vi "cbm.vi"() -> ()   [LabVIEW 2017]
uses:
  typedefs/stagestates.ctl
  typedefs/stagequeue.ctl
  typedefs/Camqueue.ctl
  typedefs/Camstates.ctl
  <vilib>/Analysis/NI_AALBase.lvlib
  <vilib>/Utility/miscctls.llb/LVMinMaxIncTypeDef.ctl
panel:
  out "white level":u16
  out "black level":u16
  out "Ranges":T2
  out "total time":u32
  out "average time per step":dbl
  out "start time":u32
  out "Stack Folder":path
  in  "Image path used":path
  in  "Save next image":bool
  out "Image":u16[][](graph)
  in  "Live Update":bool
  out "Cam ready":bool
  out "Scan points":dbl[](array[numeric])
  in  "Get mean image button":bool
  in  "Get random stack":bool
  in  "abort button":bool
  in  "Get Speckle Stack button":bool
  in  "stop button":bool
  in  "Stage position":dbl(slide) scale=-3000.0..3000.0
  in  "Tab Control":enum32{"Stage", "Camera"}(tab)
  in  "Folder Name":string
  in  "Base path":path=path "D:/Jean-Claude/180614 clem uzh"
  in  "Speckle Stack Settings":T3={"Start Position[µm]"=-150.0, "Final Position[µm]"=150.0, "Number of frames"=100} {"Number of frames" min=2; "Final Position[µm]" min=-6000.0 max=6000.0; "Start Position[µm]" min=-6000.0 max=6000.0}
  in  "Zero Ch2":bool
  out "Stage State":T4=enum."Init"
  out "Stage initialized":bool
  out "stack folder":path
  in  "settling time":u32=20
  out "size stage queue":i32
  in  "ChangeCamSettings":bool
  out "Current Settings":T5
  out "Camera Details":T6
  out "Cam state":T7
  in  "Camera index":u32
  out "Initialized":bool
  in  "use cam":bool=TRUE
  in  "input cluster":T8={"binning"=0.0, "exp. time[ms]"=100.0, "v. offset"=0, "h. offset"=0, "width"=3000, "height"=1024} {"binning" min=0.0 max=2.0 step=1.0; "v. offset" max=2048 step=4; "h. offset" max=2048 step=4; "width" max=2048 step=4; "height" max=2048 step=4}
  out "size cam queue":i32
  out "Histogram":T9(graph)
  in  "Black and White levels":cluster{u16, u16}(slide)={0, 255} scale=0.0..65535.0
  in  "scale exp":bool
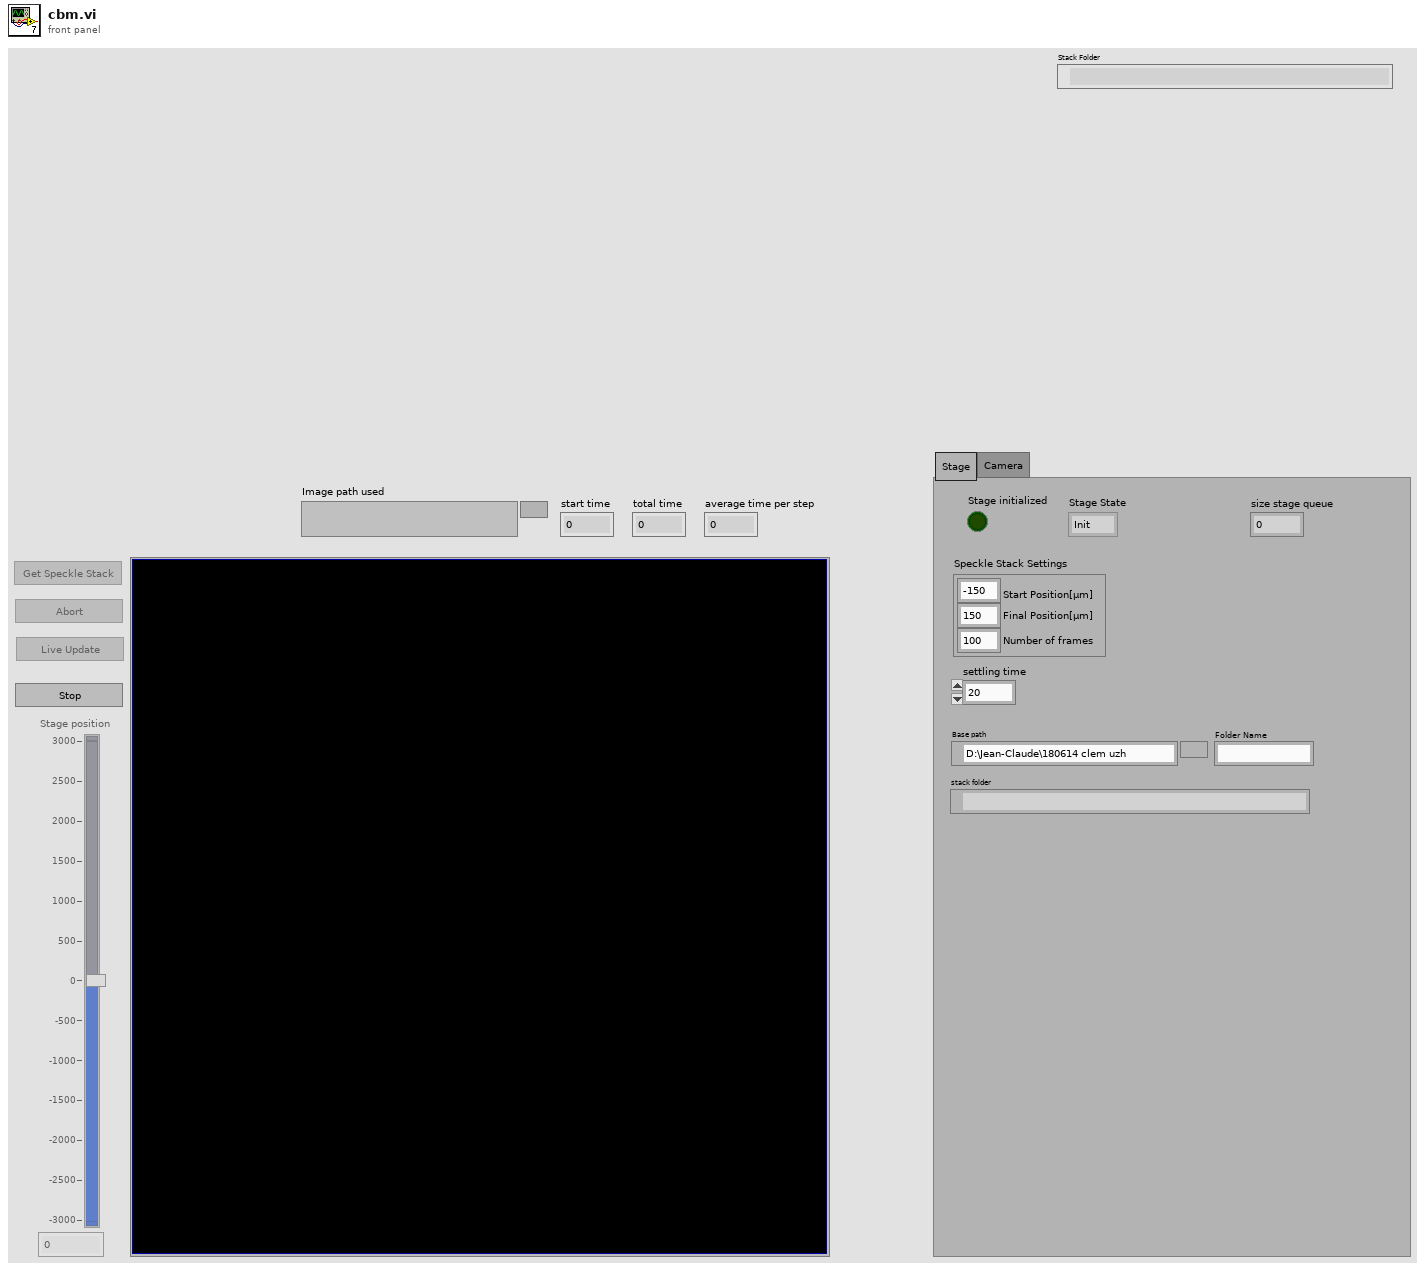
[diagram p1: front panel]
types:
  T1 = typedef "LVMinMaxIncTypeDef.ctl" = cluster{"Minimum":dbl, "Maximum":dbl, "Increment":dbl}
  T2 = cluster{"HorPosRange":T1, "VertPosRange":T1, "WidthRange":T1, "HeightRange":T1}
  T3 = cluster{"Start Position[µm]":dbl, "Final Position[µm]":dbl, "Number of frames":u32}
  T4 = typedef "stagestates.ctl" = enum16{"zero", "move", "Init", "idle", "init scan", "scan", "finish scan", "error", "stop"}
  T5 = cluster{"binning":dbl, "exposure time[s]":dbl, "v. offset":dbl, "h. offset":dbl, "width":dbl, "height":dbl}
  T6 = cluster{"Model":string, "Camera ID":string, "Firmware":string}
  T7 = typedef "Camstates.ctl" = enum16{"Intitializing", "idling", "change settings", "take snapshot", "error", "stop"}
  T8 = cluster{"binning":dbl, "exp. time[ms]":dbl, "v. offset":u32, "h. offset":u32, "width":u32, "height":u32}
  T9 = cluster{"X Values":dbl[], "Histogram: h(x)":i32[]}
  T10 = typedef "Camqueue.ctl" = enum16{"initialize camera", "Take snapshot", "Change settings", "Stop", "Scan"}
  T11 = typedef "stagequeue.ctl" = enum16{"idle", "initialize stage", "move ch2", "zero ch2", "Scan", "Stop"}
  T12 = cluster{"posX":i32, "posY":i32, "Width":i32, "height":i32}
  T13 = typedef "imagedata.ctl" = cluster{"image type":i32, "image depth":i32, "image":u8[], "mask":u8[], "colors":u32[], "Rectangle":cluster{"left":i16, "top":i16, "right":i16, "bottom":i16}}
  T14 = enum8{"Enabled", "Disabled", "Disabled and Grayed Out"}
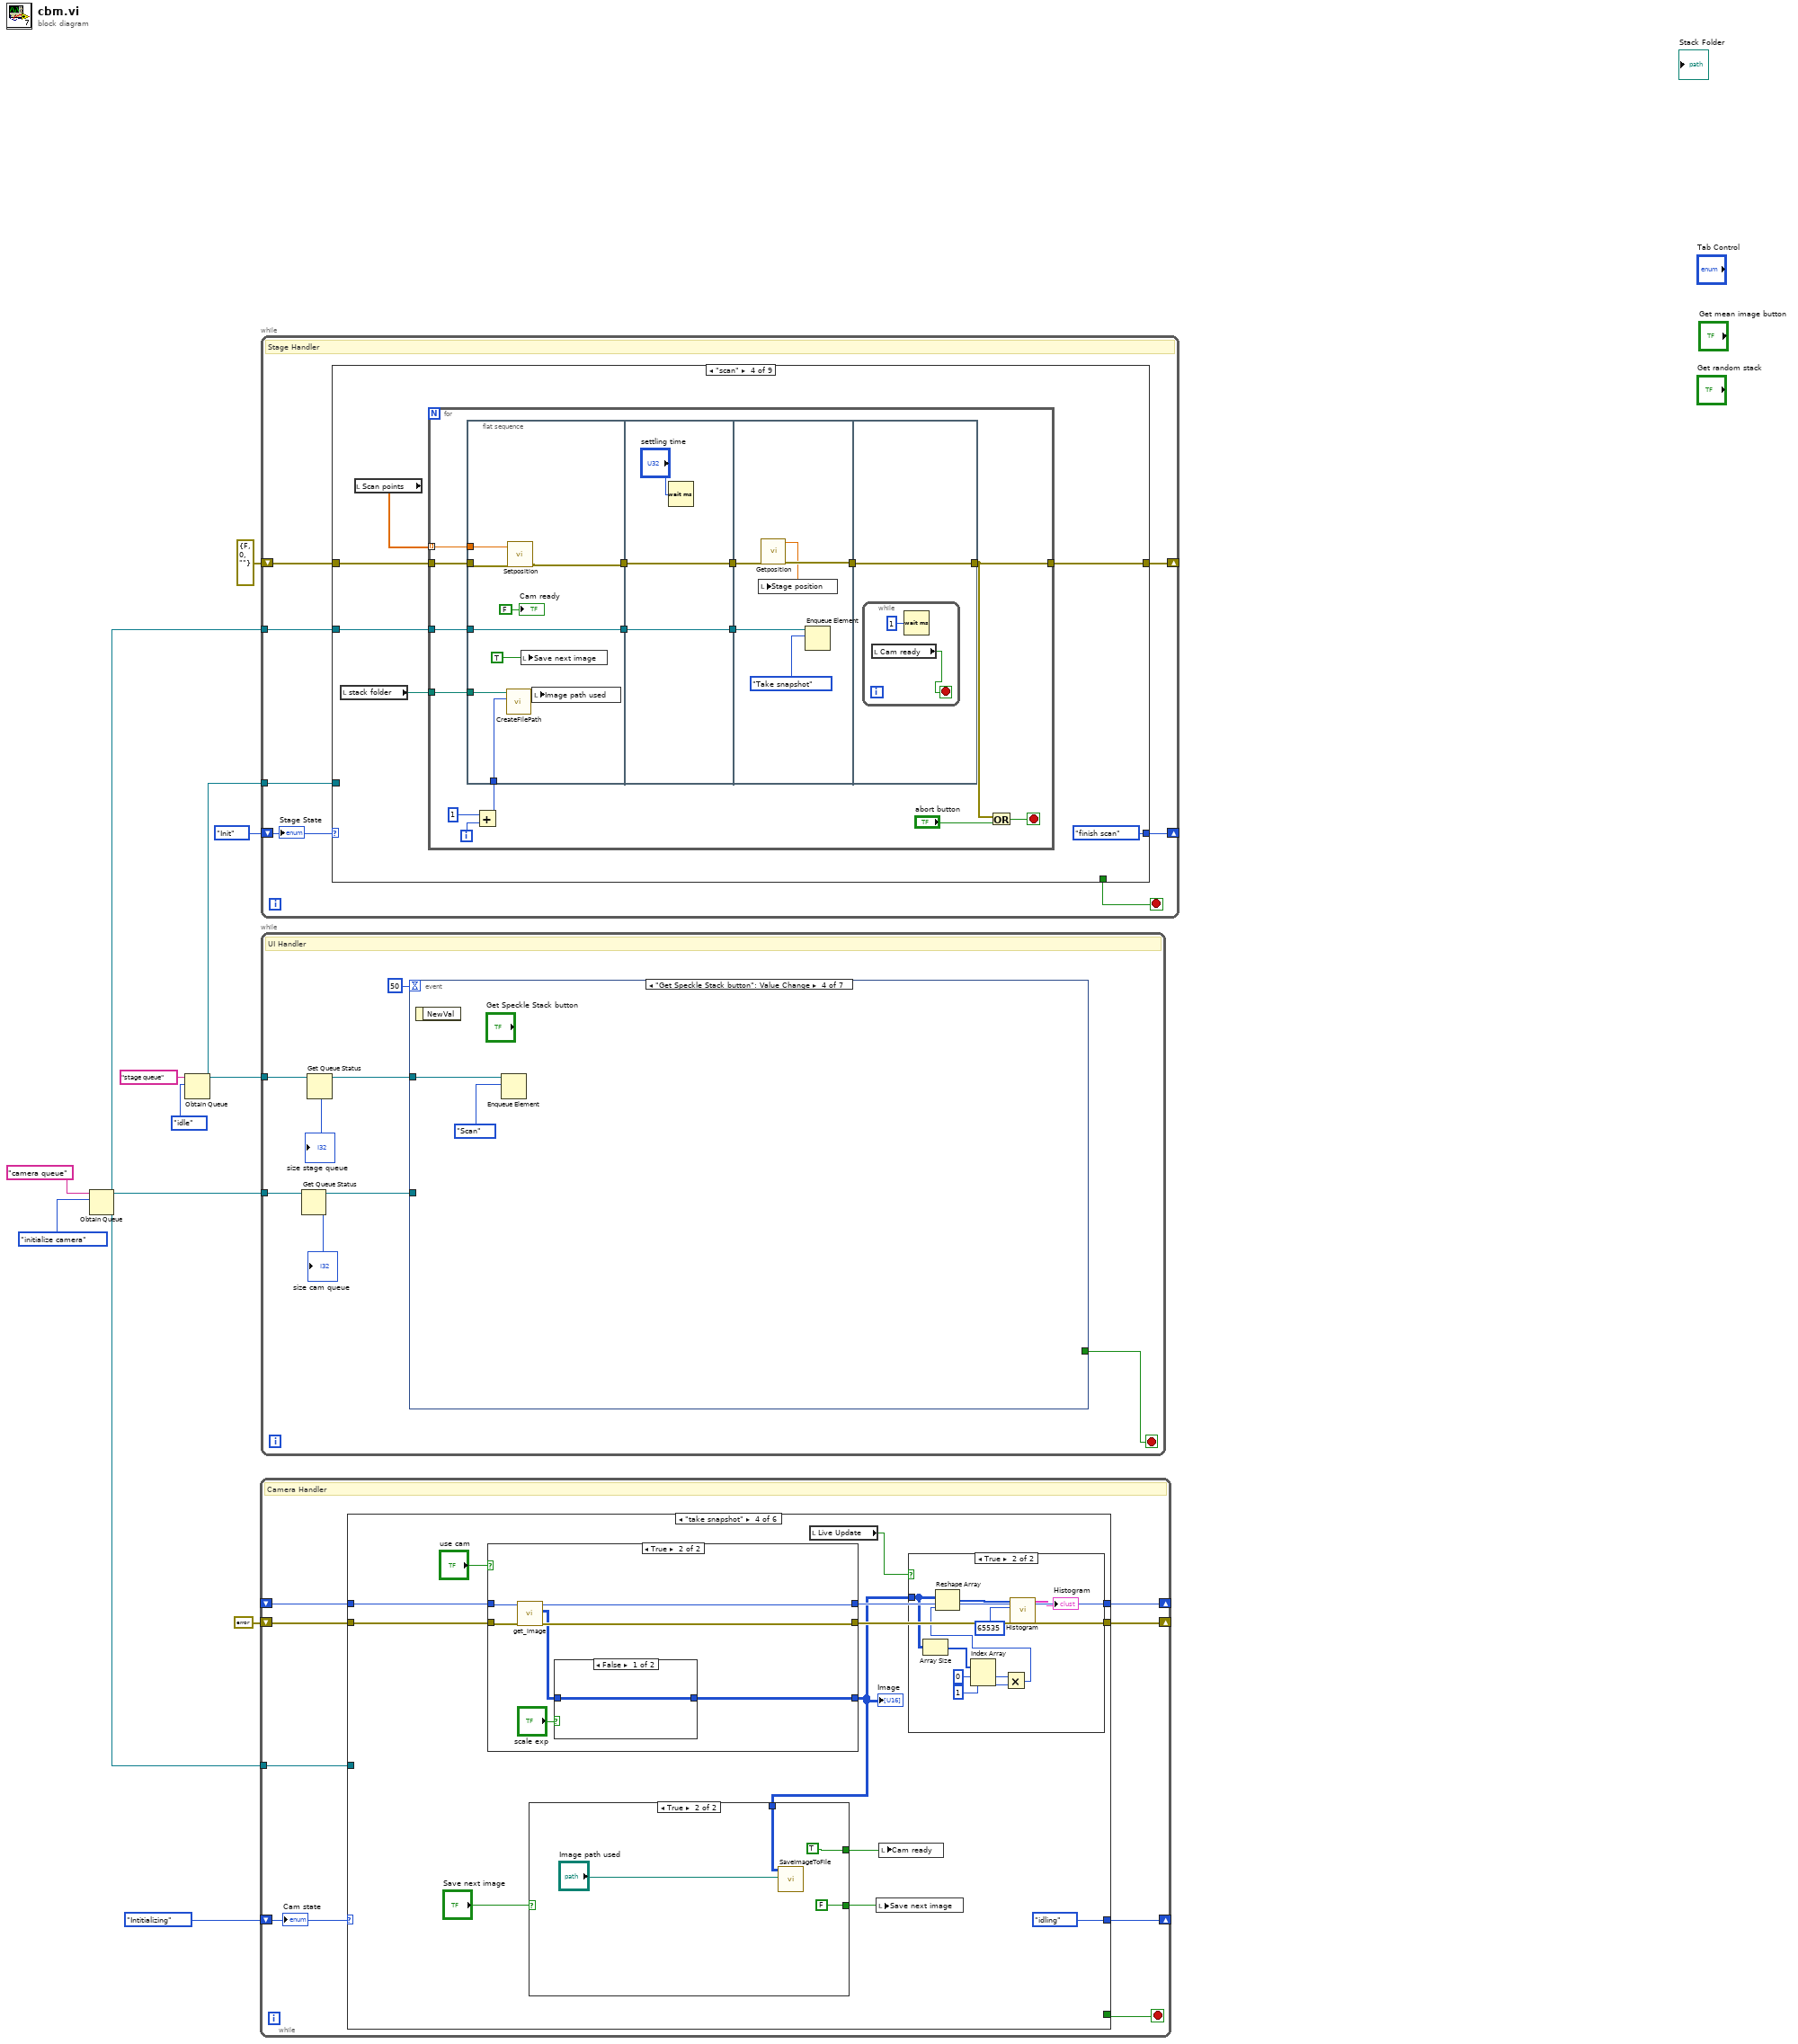
[diagram p0: block diagram]
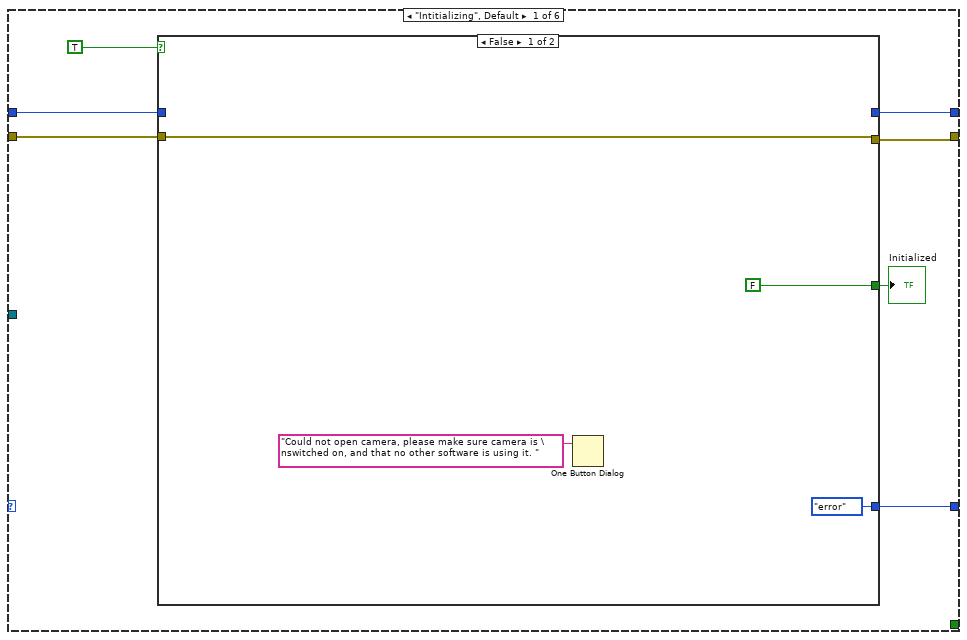
[diagram p2: hidden frame]
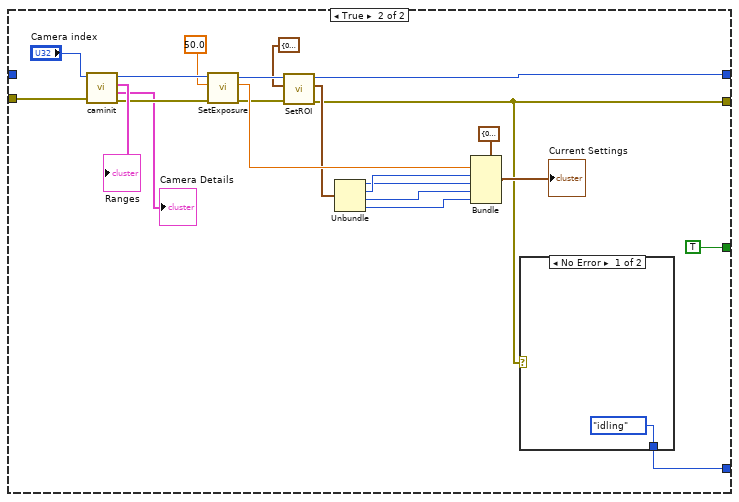
[diagram p3: hidden frame]
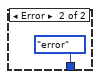
[diagram p4: hidden frame]
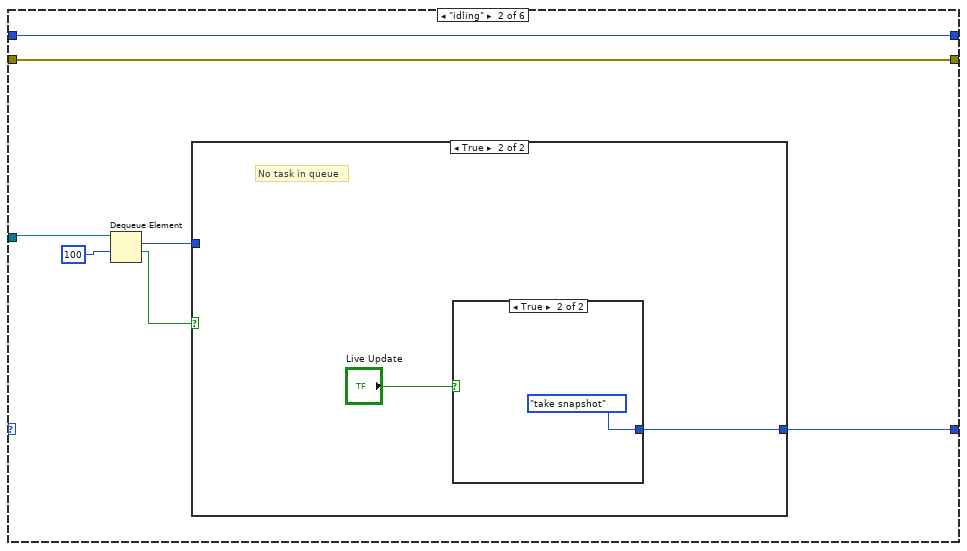
[diagram p5: hidden frame]
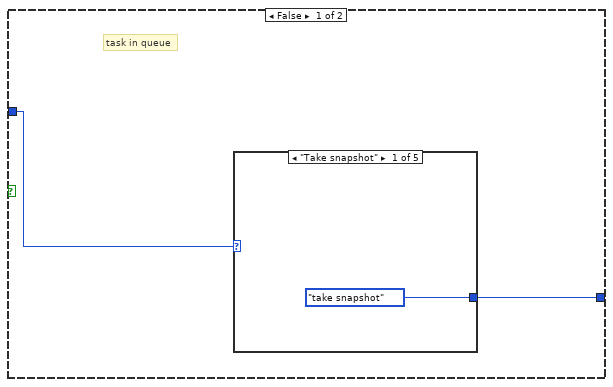
[diagram p6: hidden frame]
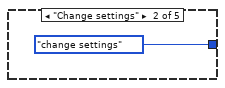
[diagram p7: hidden frame]
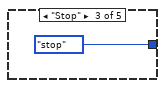
[diagram p8: hidden frame]
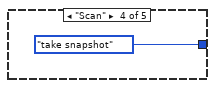
[diagram p9: hidden frame]
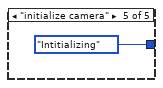
[diagram p10: hidden frame]
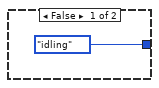
[diagram p11: hidden frame]
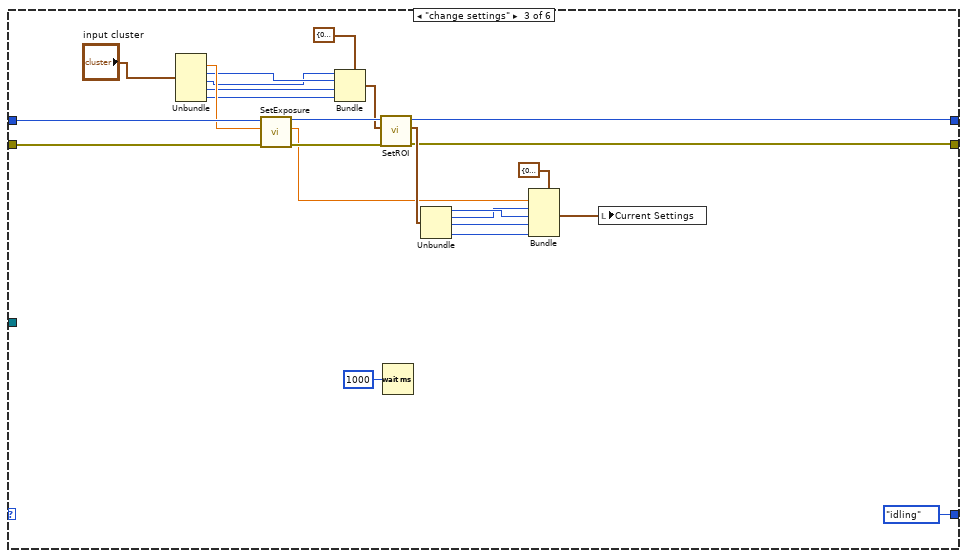
[diagram p12: hidden frame]
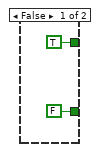
[diagram p14: hidden frame]
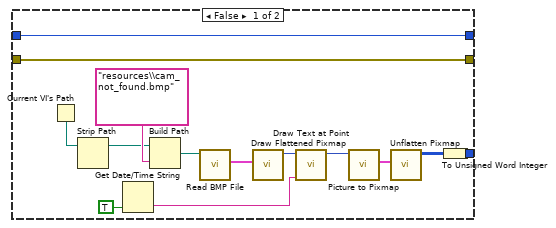
[diagram p15: hidden frame]
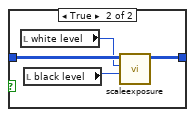
[diagram p16: hidden frame]
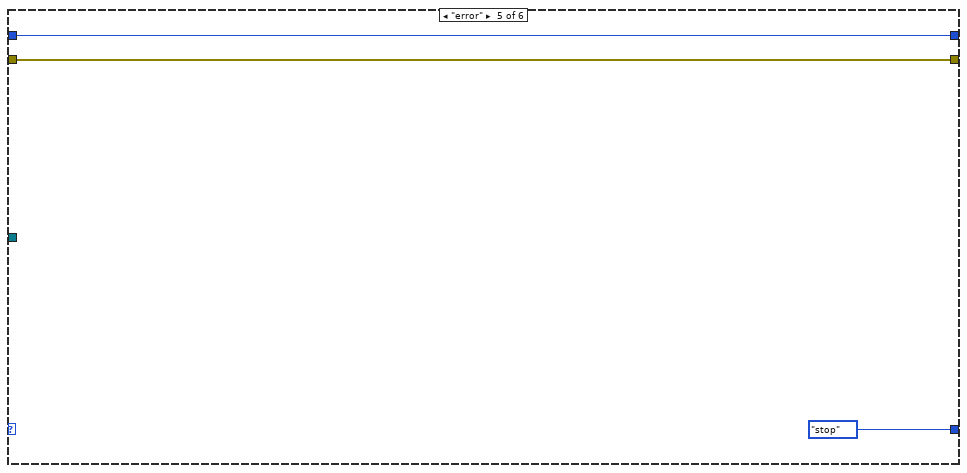
[diagram p17: hidden frame]
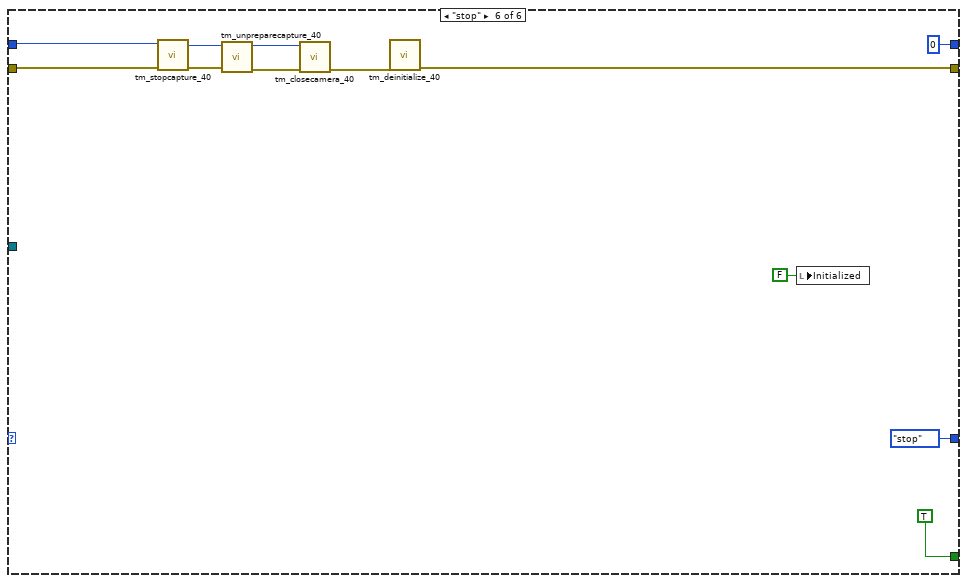
[diagram p18: hidden frame]
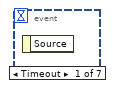
[diagram p19: hidden frame]
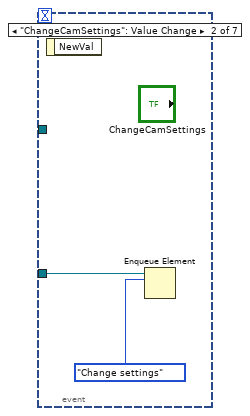
[diagram p20: hidden frame]
diagram:
  n1 = Obtain Queue(name (unnamed)="camera queue", element data type=Camqueue."initialize camera") -> (queue out=w1:refnum<queue>)  [unwired: 3 in, 2 out]
  n2 = Obtain Queue(name (unnamed)="stage queue", element data type=stagequeue."idle") -> (queue out=w5:refnum<queue>)  [unwired: 3 in, 2 out]
  n3 = while {
    tunnel: w1 -> [w11]
    shift-right: [w14] -> _
    shift-left: errorcluster {"status"=FALSE, "code"=0, "source"=""} ("error in (no error)") -> [w16]
    shift-right: [w15] -> _
    shift-left: _ -> [w12]
    shift-right: [w13] -> _
    shift-left: Camstates."Intitializing" -> [w18]
    stop <- w17 stop-if-true
    # "Camera Handler"
    n4 = case shown="\"take snapshot\"" w18 {
      tunnel: [_ _ _ _ _ TRUE] -> w17
      tunnel: w16 -> [w20 w59 w90 w104 w150 w160]
      tunnel: [w25 w60 w72 w103 w149 u32 0 ("Handle out")] -> w15
      tunnel: [w19 w59 w73 w102 w150 w156] -> w14
      tunnel: [w23 w54 Camstates."idling" Camstates."idling" Camstates."stop" Camstates."stop"] -> w13
      tunnel: w12 -> [w21 w60 w92 w105 w149 w152]
      tunnel: w11 -> [_ w58 _ _ _ _]
      frame "Intitializing", Default {
        n5 = case shown="False" TRUE {
          tunnel: [_ w40] -> w25
          tunnel: [FALSE ("Initialized") TRUE ("Initialized")] -> w24
          tunnel: [Camstates."error" w50] -> w23
          tunnel: w21 -> [_ _]
          tunnel: w20 -> [w26 w43]
          tunnel: [w26 w32] -> w19
          frame False {
            n6 = One Button Dialog(message="Could not open camera, please make sure camera is \nswitched on, and that no other software is using it. ") -> ()  [unwired: 1 in, 1 out]
          }
          frame True {
            n7 = call "caminit.vi"("error in (no error)"=w43, "Camera Index"="Camera index") -> ("error out"=w44:errorcluster, "Cam Info"=→"Camera Details":T6, "Ranges"=→"Ranges":T2, "Handle out"=w47:u32)  [unwired: 5 in]
            n8 = call "SetExposure.vi"("error in (no error)"=w44, "Exposure[ms]"=50.0, "Handle in"=w47) -> ("error out"=w33:errorcluster, "exposure"=w45:dbl, "Handle out"=w42:u32)  [unwired: 4 in, 1 out]
            n9 = call "SetROI.vi"("error in (no error)"=w33, "SizeIn"=T12 {"posX"=0, "posY"=0, "Width"=2048, "height"=2048}, "Handle in"=w42) -> ("error out"=w32:errorcluster, "sizeout"=w38:T12, "Handle out"=w40:u32)  [unwired: 5 in]
            n10 = Unbundle(w38) -> ("posX"=w36:i32, "posY"=w37:i32, "Width"=w35:i32, "height"=w34:i32)
            n11 = Bundle(cluster=T5 {"binning"=0.0, "exposure time[s]"=0.0, "v. offset"=0.0, "h. offset"=0.0, "width"=0.0, "height"=0.0} ("Current Settings"), "exposure time[s]"=w45, "v. offset"=w37, "h. offset"=w36, "width"=w35, "height"=w34) -> (→"Current Settings":T5)  [unwired: 1 in]
            n12 = case shown="No Error" w32 {
              tunnel: [Camstates."idling" Camstates."error"] -> w50
              frame No Error {
              }
              frame Error {
              }
            }
          }
        }
        "Initialized" <- w24
      }
      frame "idling" {
        n13 = Dequeue Element(queue=w58, timeout in ms (-1)=100) -> (element=w55:T10, timed out?=w56:bool)  [unwired: 1 in, 2 out]
        n14 = case shown="True" w56 {
          tunnel: w55 -> [w62 _]
          tunnel: [w61 w68] -> w54
          frame False {
            # "task in queue"
            n15 = case shown="\"Take snapshot\"" w62 {
              tunnel: [Camstates."take snapshot" Camstates."change settings" Camstates."stop" Camstates."take snapshot" Camstates."Intitializing"] -> w61
              frame "Take snapshot" {
              }
              frame "Change settings" {
              }
              frame "Stop" {
              }
              frame "Scan" {
              }
              frame "initialize camera" {
              }
            }
          }
          frame True {
            # "No task in queue"
            n16 = case shown="True" "Live Update" {
              tunnel: [Camstates."idling" Camstates."take snapshot"] -> w68
              frame False {
              }
              frame True {
              }
            }
          }
        }
      }
      frame "change settings" {
        n17 = Unbundle("input cluster") -> ("exp. time[ms]"=w91:dbl, "v. offset"=w85:u32, "h. offset"=w84:u32, "width"=w83:u32, "height"=w82:u32)  [unwired: 1 out]
        n18 = call "SetExposure.vi"("error in (no error)"=w90, "Exposure[ms]"=w91, "Handle in"=w92) -> ("error out"=w88:errorcluster, "exposure"=w78:dbl, "Handle out"=w89:u32)  [unwired: 4 in, 1 out]
        n19 = Bundle(cluster=T12 {"posX"=0, "posY"=0, "Width"=0, "height"=0} ("SizeIn"), "posX"=w84, "posY"=w85, "Width"=w83, "height"=w82) -> (w86:T12)
        n20 = call "SetROI.vi"("error in (no error)"=w88, "SizeIn"=w86, "Handle in"=w89) -> ("error out"=w73:errorcluster, "sizeout"=w79:T12, "Handle out"=w72:u32)  [unwired: 5 in]
        n21 = Wait (ms)(milliseconds to wait=u32 1000) -> ()  [unwired: 1 out]
        n22 = Unbundle(w79) -> ("posX"=w77:i32, "posY"=w76:i32, "Width"=w75:i32, "height"=w74:i32)
        n23 = Bundle(cluster=T5 {"binning"=0.0, "exposure time[s]"=0.0, "v. offset"=0.0, "h. offset"=0.0, "width"=0.0, "height"=0.0} ("Current Settings"), "exposure time[s]"=w78, "v. offset"=w76, "h. offset"=w77, "width"=w75, "height"=w74) -> (w80:T5)  [unwired: 1 in]
        n24 = local write "Current Settings"(w80) -> ()
      }
      frame "take snapshot" {
        n25 = case shown="True" "use cam" {
          tunnel: w104 -> [w132 w143]
          tunnel: [w132 w142] -> w102
          tunnel: [w131 w140] -> w103
          tunnel: w105 -> [w131 w141]
          tunnel: [w123 w138] -> w96
          frame False {
            n26 = Current VI's Path() -> (path=w136:path)
            n27 = Strip Path(path=w136) -> (stripped path=w134:path)  [unwired: 1 out]
            n28 = Get Date/Time String(want seconds? (F)=TRUE) -> (time string=w128:string)  [unwired: 2 in, 1 out]
            n29 = Build Path(base path=w134, name or relative path="resources\\cam_not_found.bmp") -> (appended path=w133:path)
            n30 = call <vilib>:"Read BMP File.vi"("path to BMP file"=w133) -> ("image data"=w130:T13)  [unwired: 8 in, 2 out]
            n31 = call <vilib>:"Draw Flattened Pixmap.vi"("image data"=w130) -> ("new picture"=w129:picture)  [unwired: 8 in]
            n32 = call <vilib>:"Draw Text at Point.vi"("text"=w128, "picture"=w129) -> ("new picture"=w127:picture)  [unwired: 8 in, 1 out]
            n33 = call <vilib>:"Picture to Pixmap.vi"("picture"=w127) -> ("image data"=w126:T13)  [unwired: 9 in, 1 out]
            n34 = call <vilib>:"Unflatten Pixmap.vi"("image data"=w126) -> ("24-bit pixmap"=w124:u32[][])  [unwired: 4 in, 6 out]
            n35 = To Unsigned Word Integer(number=w124) -> (unsigned 16bit integer=w123:u16[][])
          }
          frame True {
            n36 = call "get_image.vi"("error in (no error)"=w143, "Handle in"=w141) -> ("error out"=w142:errorcluster, "Data"=w139:u16[][], "Handle out"=w140:u32)  [unwired: 7 in]
            n37 = case shown="False" "scale exp" {
              tunnel: w139 -> [w144 w148]
              tunnel: [w144 w147] -> w138
              frame False {
              }
              frame True {
                n38 = local read "white level"() -> (w146:u16)
                n39 = local read "black level"() -> (w145:u16)
                n40 = call "scaleexposure.vi"("black"=w145, "white"=w146, "image in"=w148) -> ("image out"=w147:u16[][])  [unwired: 8 in]
              }
            }
          }
        }
        "Image" <- w96
        n41 = case shown="True" "Save next image" {
          tunnel: [FALSE ("Save next image") FALSE ("Save next image")] -> w100
          tunnel: [TRUE TRUE] -> w99
          tunnel: w96 -> [_ w119]
          frame False {
          }
          frame True {
            n42 = call "SaveImageToFile.vi"("File Path"="Image path used", "Image Pixels (U16)"=w119) -> ()  [unwired: 9 in, 1 out]
          }
        }
        n43 = local read "Live Update"() -> (w97:bool)
        n44 = local write "Save next image"(w100) -> ()
        n45 = local write "Cam ready"(w99) -> ()
        n46 = case shown="True" w97 {
          tunnel: w96 -> [_ w115]
          frame False {
          }
          frame True {
            n47 = Array Size(array=w115) -> (size(s)=w112:i32[])
            n48 = Index Array(array=w112, index #1=0 ("index"), index #2=1 ("index")) -> (element #1=w111:i32, element #2=w110:i32)
            n49 = Multiply(x=w111, y=w110) -> (x*y=w109:i32)
            n50 = Reshape Array(w115, w109) -> (w116:u16[])
            n51 = call <vilib>:"Histogram.vi"("intervals"=65535, "X"=w116) -> ("Histogram Graph"=→"Histogram":T9)  [unwired: 6 in, 3 out]
          }
        }
      }
      frame "error" {
      }
      frame "stop" {
        n52 = call <userlib>:"tm_stopcapture_40.vi"("error in (no error)"=w160, "Handle in"=w152) -> ("error out"=w159:errorcluster, "Handle out"=w153:u32)  [unwired: 8 in]
        n53 = call <userlib>:"tm_unpreparecapture_40.vi"("error in (no error)"=w159, "Handle in"=w153) -> ("error out"=w158:errorcluster, "Handle out"=w154:u32)  [unwired: 8 in]
        n54 = call <userlib>:"tm_closecamera_40.vi"("error in (no error)"=w158, "Handle in"=w154) -> ("error out"=w157:errorcluster)  [unwired: 9 in]
        n55 = call <userlib>:"tm_deinitialize_40.vi"("error in (no error)"=w157) -> ("error out"=w156:errorcluster)  [unwired: 10 in]
        n56 = local write "Initialized"(FALSE ("Initialized")) -> ()
      }
    }
    "Cam state" <- w18
  }
  n57 = while {
    shift-right: [w169] -> _
    shift-left: stagestates."Init" -> [w170]
    shift-right: [w168] -> _
    shift-left: errorcluster {"status"=FALSE, "code"=0, "source"=""} ("error out") -> [w167]
    tunnel: w5 -> [w165]
    tunnel: w1 -> [w164]
    stop <- w166 stop-if-true
    # "Stage Handler"
    n58 = case shown="\"scan\"" w170 {
      tunnel: [w174 w187 stagestates."scan" stagestates."finish scan" stagestates."idle" stagestates."Init" stagestates."stop" stagestates."idle" stagestates."idle"] -> w169
      tunnel: [w171 w184 w221 w235 w281 w286 w297 w302 w306] -> w168
      tunnel: w167 -> [w172 w185 w221 w236 w281 w289 w298 w303 w306]
      tunnel: [FALSE FALSE FALSE _ _ _ TRUE _ _] -> w166
      tunnel: w165 -> [_ w191 _ _ _ _ _ _ _]
      tunnel: w164 -> [_ _ _ w234 _ _ _ _ _]
      frame "Init", Default {
        n59 = call "init.vi"("error in"=w172, "Controller S/N"="118032250") -> ("error out"=w171:errorcluster)  [unwired: 9 in]
        n60 = case shown="No Error" w171 {
          tunnel: [stagestates."error" stagestates."idle"] -> w174
          tunnel: [FALSE ("Stage initialized") TRUE ("Stage initialized")] -> w176
          frame Error {
            n61 = Wait (ms)(milliseconds to wait=u32 10000) -> ()  [unwired: 1 out]
          }
          frame No Error {
            w180 = T14."Enabled" ("Disabled")
            n62 = property on="Stage position" class="Slide (strict)"("DisabledEnum"=w180) -> ()  [unwired: 2 in, 2 out]
            n63 = property on="Get Speckle Stack button" class="Bool"("DisabledEnum"=w180) -> ()  [unwired: 2 in, 2 out]
            n64 = property on="Get mean image button" class="Bool"("DisabledEnum"=w180) -> ()  [unwired: 2 in, 2 out]
            n65 = property on="Get random stack" class="Bool"("DisabledEnum"=w180) -> ()  [unwired: 2 in, 2 out]
            n66 = property on="abort button" class="Bool"("DisabledEnum"=w180) -> ()  [unwired: 2 in, 2 out]
            n67 = property on="Live Update" class="Bool (strict)"("DisabledEnum"=w180) -> ()  [unwired: 2 in, 2 out]
          }
        }
        "Stage initialized" <- w176
      }
      frame "idle" {
        n68 = Dequeue Element(queue=w191, timeout in ms (-1)=20) -> (element=w189:T11, timed out?=w188:bool)  [unwired: 1 in, 2 out]
        n69 = case shown="True" w188 {
          tunnel: w189 -> [w194 _]
          tunnel: [w193 stagestates."idle"] -> w186
          frame False {
            # "Queue not empty"
            n70 = case shown="\"zero ch2\"" w194 {
              tunnel: [stagestates."idle" stagestates."Init" stagestates."move" stagestates."zero" stagestates."init scan" stagestates."stop"] -> w193
              frame "idle", Default {
              }
              frame "initialize stage" {
              }
              frame "move ch2" {
              }
              frame "zero ch2" {
              }
              frame "Scan" {
              }
              frame "Stop" {
              }
            }
          }
          frame True {
            # "Queue empty"
          }
        }
        n71 = call "Getposition.vi"("error in"=w185) -> ("error out"=w184:errorcluster, "Position[µm]"=w183:dbl)  [unwired: 9 in]
        n72 = case shown="No Error" w184 {
          tunnel: [stagestates."error" w203] -> w187
          tunnel: w183 -> [_ _]
          tunnel: w186 -> [_ w203]
          frame Error {
          }
          frame No Error {
          }
        }
      }
      frame "init scan" {
        n73 = Unbundle("Speckle Stack Settings") -> ("Start Position[µm]"=w208:dbl, "Final Position[µm]"=w209:dbl, "Number of frames"=w217:u32)
        n74 = Subtract(x=w217, y=u32 1) -> (x-y=w214:u32)
        n75 = Subtract(x=w209, y=w208) -> (x-y=w218:dbl)
        n76 = Divide(x=w218, y=w214) -> (x/y=w216:dbl)
        n77 = property on="Stage position" class="Slide (strict)"("DisabledEnum"=T14."Disabled and Grayed Out" ("Disabled")) -> ()  [unwired: 2 in, 2 out]
        n78 = property on="Live Update" class="Bool (strict)"("Value"=FALSE ("abort button"), "DisabledEnum"=T14."Disabled and Grayed Out" ("Disabled")) -> ()  [unwired: 2 in, 2 out]
        n79 = while {
          tunnel: w208 -> [w231]
          tunnel: w216 -> [w230]
          shift-right: [w226] -> w213
          shift-left: dbl[] [] -> [w227]
          tunnel: w214 -> [w224]
          i -> [w225]
          stop <- w229 stop-if-true
          n80 = Multiply(x=w230, y=w225) -> (x*y=w232:dbl)
          n81 = Add(x=w231, y=w232) -> (x+y=w228:dbl)
          n82 = Equal?(x=w225, y=w224) -> (x = y?=w229:bool)
          n83 = Build Array (concatenate)(w227, w228) -> (w226:dbl[])
        }
        "Scan points" <- w213
        n84 = call "createfolderincrementing.vi"("Base path"="Base path", "Folder Name"="Folder Name") -> ("created path"=→"stack folder":path)  [unwired: 8 in, 1 out]
        n85 = Tick Count (ms)() -> (millisecond timer value=→"start time":u32)
      }
      frame "scan" {
        n86 = local read "stack folder"() -> (w233:path)
        n87 = local read "Scan points"() -> (w237:dbl[])
        n88 = for {
          tunnel: w237 -> [w252] mode=indexing
          tunnel: w236 -> [w253]
          tunnel: [w244] -> w235
          tunnel: w234 -> [w250]
          tunnel: w233 -> [w247]
          i -> [w249]
          stop <- w243 stop-if-true
          n89 = flat-sequence {
            tunnel: w253 -> [w255]
            tunnel: w252 -> [w254]
            tunnel: [w256] -> w242
            tunnel: [w261] -> w240
            tunnel: w250 -> [w261]
            tunnel: w247 -> [w259]
            tunnel: w246 -> [w260]
            tunnel: w242 -> [w265]
            tunnel: [w265] -> w241
            tunnel: w240 -> [w264]
            tunnel: [w264] -> w239
            tunnel: w241 -> [w268]
            tunnel: [w267] -> w251
            tunnel: w239 -> [w269]
            tunnel: w251 -> [w271]
            tunnel: [w271] -> w244
            frame #0 {
              n90 = call "CreateFilePath.vi"("Frame number"=w260, "folder"=w259) -> ("Path to file"=w258:path)  [unwired: 9 in]
              n91 = call "Setposition.vi"("error in"=w255, "Position[µm]"=w254) -> ("error out"=w256:errorcluster)  [unwired: 9 in]
              n92 = local write "Save next image"(TRUE ("Save next image")) -> ()
              n93 = local write "Image path used"(w258) -> ()
              "Cam ready" <- FALSE ("Camera ready")
            }
            frame #1 {
              n94 = Wait (ms)(milliseconds to wait="settling time") -> ()  [unwired: 1 out]
            }
            frame #2 {
              n95 = call "Getposition.vi"("error in"=w268) -> ("error out"=w267:errorcluster, "Position[µm]"=w266:dbl)  [unwired: 9 in]
              n96 = local write "Stage position"(w266) -> ()
              n97 = Enqueue Element(queue=w269, element=Camqueue."Take snapshot") -> ()  [unwired: 2 in, 3 out]
            }
            frame #3 {
              n98 = while {
                stop <- w273 stop-if-true
                n99 = local read "Cam ready"() -> (w273:bool)
                n100 = Wait (ms)(milliseconds to wait=u32 1) -> ()  [unwired: 1 out]
              }
            }
          }
          n101 = Add(x=1, y=w249) -> (x+y=w246:i32)
          n102 = Or(x=w244, y="abort button") -> (x .or. y?=w243:bool)
        }
      }
      frame "finish scan" {
        w280 = T14."Enabled" ("Disabled")
        n103 = property on="Live Update" class="Bool (strict)"("Value"=FALSE ("abort button"), "DisabledEnum"=w280) -> ()  [unwired: 2 in, 2 out]
        n104 = property on="Stage position" class="Slide (strict)"("DisabledEnum"=w280) -> ()  [unwired: 2 in, 2 out]
        n105 = local read "start time"() -> (w274:u32)
        n106 = Tick Count (ms)() -> (millisecond timer value=w275:u32)
        n107 = property on="Number of frames" class="DigNum (strict)"() -> ("Value"=w276:u32)  [unwired: 2 in, 2 out]
        n108 = Subtract(x=w275, y=w274) -> (x-y=w278:u32)
        "total time" <- w278
        n109 = Divide(x=w278, y=w276) -> (x/y=→"average time per step":dbl)
      }
      frame "error" {
        n110 = call "ERR?.vi"("error in"=w289) -> ("error out"=w288:errorcluster)  [unwired: 1 in, 17 out]
        n111 = call "GCSTranslateError.vi"("error in"=w288) -> ("Error Description"=w287:string, "error out"=w285:errorcluster)  [unwired: 17 out]
        n112 = Concatenate Strings("An error with the stage occurred in function:\\n" ("message"), w287, "\\n\nwill atttempt to reinitialize" ("string")) -> (w291:string)
        n113 = One Button Dialog(message=w291) -> ()  [unwired: 1 in, 1 out]
        n114 = property on="Stage position" class="Slide (strict)"("Value"=0.0 ("Ch2_control"), "DisabledEnum"=T14."Disabled and Grayed Out" ("Disabled")) -> ()  [unwired: 2 in, 2 out]
        n115 = call "Close connection if open.vi"("System no."=1, "error in"=w285) -> ("error out"=w284:errorcluster)  [unwired: 1 in, 16 out]
        n116 = call <vilib>:"Clear Errors.vi"("error in (no error)"=w284) -> ("error out"=w286:errorcluster)  [unwired: 5 in, 1 out]
      }
      frame "stop" {
        w296 = T14."Disabled and Grayed Out" ("Disabled")
        n117 = call "close.vi"("error in"=w298) -> ("error out"=w297:errorcluster)  [unwired: 10 in]
        n118 = property on="Stage position" class="Slide (strict)"("DisabledEnum"=w296) -> ()  [unwired: 2 in, 2 out]
        n119 = property on="Get random stack button" class="Bool"("DisabledEnum"=w296) -> ()  [unwired: 2 in, 2 out]
        n120 = property on="Get Speckle Stack button" class="Bool"("DisabledEnum"=w296) -> ()  [unwired: 2 in, 2 out]
        n121 = property on="Live Update" class="Bool (strict)"("DisabledEnum"=w296) -> ()  [unwired: 2 in, 2 out]
        n122 = property on="Get mean image button" class="Bool"("DisabledEnum"=w296) -> ()  [unwired: 2 in, 2 out]
        n123 = property on="abort button" class="Bool"("DisabledEnum"=w296) -> ()  [unwired: 2 in, 2 out]
        n124 = property on="Stage initialized" class="Bool (strict)"("Value"=FALSE ("Stage initialized")) -> ()  [unwired: 2 in, 2 out]
      }
      frame "move" {
        n125 = local read "Stage position"() -> (w304:dbl)
        n126 = call "Setposition.vi"("error in"=w303, "Position[µm]"=w304) -> ("error out"=w302:errorcluster)  [unwired: 9 in]
      }
      frame "zero" {
      }
    }
    "Stage State" <- w170
  }
  n127 = while {
    tunnel: w5 -> [w315]
    tunnel: w1 -> [w310]
    stop <- w314 stop-if-true
    # "UI Handler"
    n128 = Get Queue Status(queue=w310) -> (queue out=w309:refnum<queue>, # elements in queue=→"size cam queue":i32)  [unwired: 2 in, 6 out]
    n129 = Get Queue Status(queue=w315) -> (queue out=w313:refnum<queue>, # elements in queue=→"size stage queue":i32)  [unwired: 2 in, 6 out]
    n130 = event shown="[3] \"Get Speckle Stack button\": Value Change" {
      selector: _ -> [_ _ _ _ _ _ _]
      dyn-events: _ -> [_ _ _ _ _ _ _]
      timeout: 50 -> [_ _ _ _ _ _ _]
      tunnel: w313 -> [_ _ _ w324 w326 w330 w334]
      tunnel: [_ _ _ _ _ "stop button" _] -> w314
      tunnel: w309 -> [_ w317 _ _ _ w328 _]
      event Timeout {
        n131 = event-data() -> ()  [unwired: 1 in, 1 out]
      }
      event "ChangeCamSettings": Value Change {
        n132 = event-data() -> ()  [unwired: 1 in, 1 out]
        n133 = Enqueue Element(queue=w317, element=Camqueue."Change settings") -> ()  [unwired: 2 in, 3 out]
      }
      event "Black and White levels": Value Change {
        n134 = event-data() -> ("NewVal"=w322:cluster{u16, u16})  [unwired: 1 in, 5 out]
        n135 = Unbundle(w322) -> (w321:u16, w320:u16)
        n136 = Max & Min(x=w321, y=w320) -> (max(x,y)=→"white level":u16, min(x,y)=→"black level":u16)
      }
      event "Get Speckle Stack button": Value Change {
        n137 = event-data() -> ()  [unwired: 1 in, 1 out]
        n138 = Enqueue Element(queue=w324, element=stagequeue."Scan") -> ()  [unwired: 2 in, 3 out]
      }
      event "Zero Ch2": Value Change {
        n139 = event-data() -> ()  [unwired: 1 in, 1 out]
        n140 = Enqueue Element(queue=w326, element=stagequeue."zero ch2") -> ()  [unwired: 2 in, 3 out]
      }
      event "stop button": Value Change {
        n141 = event-data() -> ()  [unwired: 1 in, 2 out]
        n142 = Enqueue Element(queue=w328, element=Camqueue."Stop") -> ()  [unwired: 2 in, 3 out]
        n143 = Enqueue Element(queue=w330, element=stagequeue."Stop") -> ()  [unwired: 2 in, 3 out]
      }
      event "Stage position": Value Change {
        n144 = event-data() -> ()  [unwired: 1 in, 2 out]
        n145 = Enqueue Element(queue=w334, element=stagequeue."move ch2") -> ()  [unwired: 2 in, 3 out]
        n146 = Wait (ms)(milliseconds to wait=u32 50) -> ()  [unwired: 1 out]
      }
    }
  }
